vi "Stop Selected.vi"(8 "error in (no error)":errorcluster, 10 "index":i32, 11 "VacuumLines in":refnum<class "VacuumLines.lvclass">) -> (0 "error out":errorcluster, 3 "VacuumLines out":refnum<class "VacuumLines.lvclass">)   [LabVIEW 2016, in "Hardware.lvlib" / "VacuumLine.lvlib" / "VacuumLines.lvclass"]
uses:
  <userlib>/Common Components/Hardware/Abstract System/VacuumLine/VacuumLines/VacuumLines.lvclass
  <userlib>/Common Components/Hardware/Abstract System/VacuumLine/VacuumLines/VacuumLines.lvclass/VacuumLines.ctl
  <userlib>/Common Components/Hardware/Abstract System/VacuumLine/VacuumLine/VacuumLine.lvclass
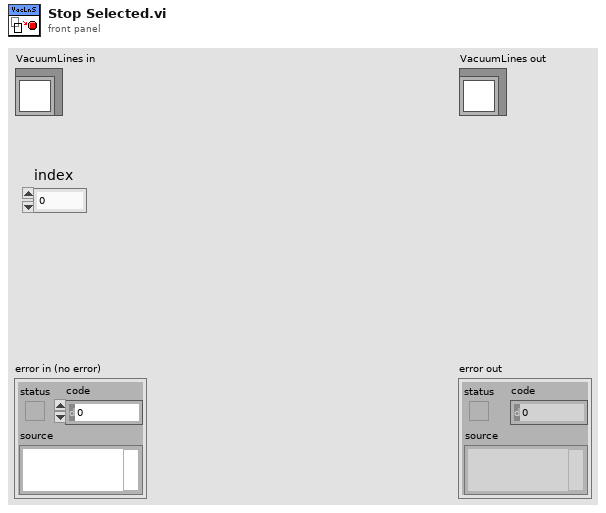
[diagram p1: front panel]
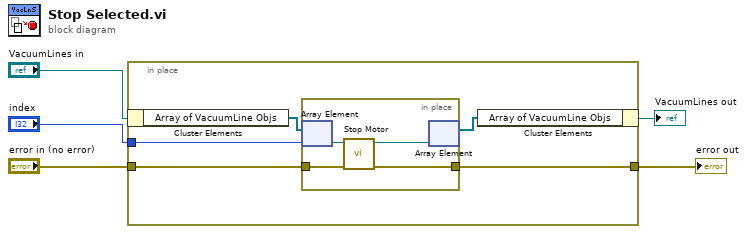
[diagram p0: block diagram]
diagram:
  n1 = in-place {
    in-place-border: "index" -> [w9]
    in-place-border: "error in (no error)" -> [w8]
    in-place-border: [w6] -> w1
    n2 = in-place-cluster #1("VacuumLines in") -> ("Array of VacuumLine Objs"=w10:refnum<class "VacuumLine.lvclass">[])
    n3 = in-place {
      in-place-border: w8 -> [w14]
      in-place-border: [w11] -> w6
      n4 = in-place-array #2(w10, w9) -> (w13:refnum<class "VacuumLine.lvclass">)
      n5 = call <userlib>:"Stop Motor.vi"("error in (no error)"=w14, "VacuumLine in"=w13) -> ("error out"=w11:errorcluster, "VacuumLine out"=w12:refnum<class "VacuumLine.lvclass">)  [unwired: 8 in]
      n6 = in-place-array #2(w12) -> (w7:refnum<class "VacuumLine.lvclass">[])  [unwired: 1 out]
    }
    n7 = in-place-cluster #1("Array of VacuumLine Objs"=w7) -> (→"VacuumLines out":refnum<class "VacuumLines.lvclass">)
  }
  "error out" <- w1
